vi "write_sync_attributes.vi"(8 "error in (no error)":errorcluster, 10 "Hydraharp Settings.Sync Settings":T1 {"snc_offs" min=-99999 max=99999 step=1; "snc_ZeroX" min=0 max=20 step=1; "snc_level" min=0 max=800 step=10}, 11 "HDF5 Ref":T3) -> (0 "error out":errorcluster, 3 "HDF5 Ref out":T3)   [LabVIEW 2015, in "hdf5_photon_record_log.lvclass"]
uses:
  hdf5_photon_record_log.lvclass
  <vilib>/UPVI/lvhdf5/library.llb/HDF5 Ref.ctl
  hydraharp_panel/hpanel_sync_settings.ctl
  hydraharp_panel/hpanel_sync_div.ctl
  <vilib>/UPVI/lvhdf5/attribute.llb/Write Multiple Attributes.vi
  <vilib>/UPVI/lvhdf5/attribute.llb/LVH5A Operation.ctl
  <vilib>/UPVI/lvhdf5/attribute.llb/LVH5 Write Attributes.xnode
  <vilib>/Utility/VariantDataType/GetClusterInfo.vi
  <vilib>/Utility/VariantDataType/VariantType.lvlib
  <vilib>/Utility/VariantDataType/GetTypeInfo.vi
  <vilib>/UPVI/lvhdf5/attribute.llb/Cluster to Attribute Array.xnode
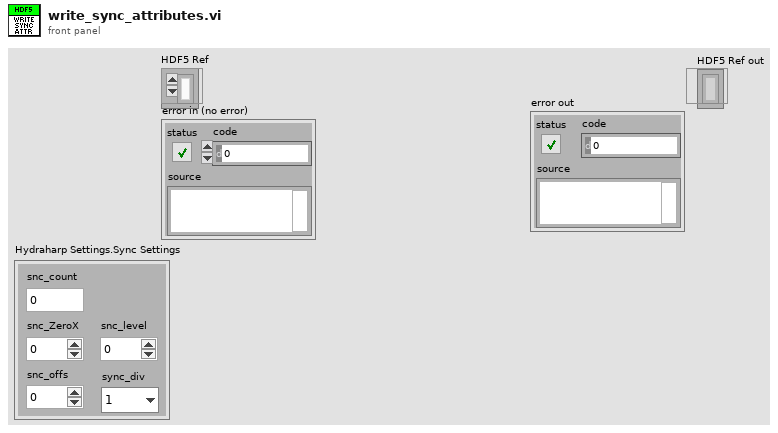
[diagram p1: front panel]
types:
  T1 = typedef "hpanel_sync_settings.ctl" = cluster{"snc_count":i32, "snc_level":i32, "snc_ZeroX":i32, "snc_offs":i32, "sync_div":T2}
  T2 = typedef "hpanel_sync_div.ctl" = enum16{"1", "2", "4", "8"}
  T3 = typedef "HDF5 Ref.ctl" = refnum<k1>
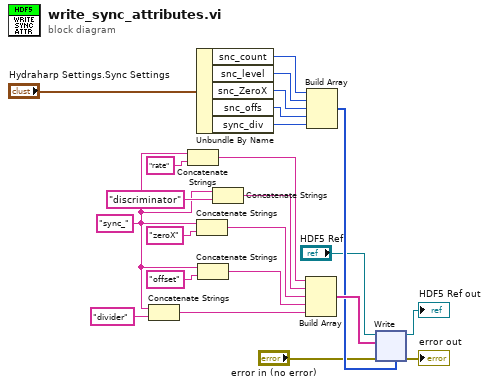
[diagram p0: block diagram]
diagram:
  w3 = "sync_" ("string")
  n1 = Concatenate Strings(w3, "divider" ("string")) -> (w7:string)
  n2 = Concatenate Strings(w3, "rate" ("string")) -> (w1:string)
  n3 = Unbundle By Name("Hydraharp Settings.Sync Settings") -> ("snc_count"=w4:i32, "snc_level"=w17:i32, "snc_ZeroX"=w16:i32, "snc_offs"=w15:i32, "sync_div"=w5:T2)
  n4 = Concatenate Strings(w3, "zeroX" ("string")) -> (w20:string)
  n5 = Concatenate Strings(w3, "offset" ("string")) -> (w19:string)
  n6 = Concatenate Strings(w3, "discriminator" ("string")) -> (w21:string)
  n7 = Build Array(w1, w21, w20, w19, w7) -> (w18:string[])
  n8 = Build Array(w4, w17, w16, w15, w5) -> (w14:i32[])
  n9 = xnode "Write"("HDF5 Ref"="HDF5 Ref", "error in (no error)"="error in (no error)", "Name(s)"=w18, "Value(s)"=w14) -> ("HDF5 Ref out"=→"HDF5 Ref out":T3, "error out"=→"error out":errorcluster)  [unwired: 1 in]
